vi "SID_mem_to_filter.vi"(11 "mem":u8[](array[numeric]) format="%02x") -> (2 "filter reg":T1 {"vol" format="%0.2f"; "res" format="%0.2f"; "freq" format="%0.2f"})   [LabVIEW 2018]
uses:
  SID_filter_reg.ctl
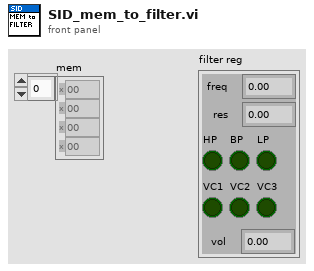
[diagram p1: front panel]
types:
  T1 = typedef "SID_filter_reg.ctl" = cluster{"freq":dbl, "res":dbl, "HP":bool, "BP":bool, "LP":bool, "VC1":bool, "VC2":bool, "VC3":bool, "vol":dbl}
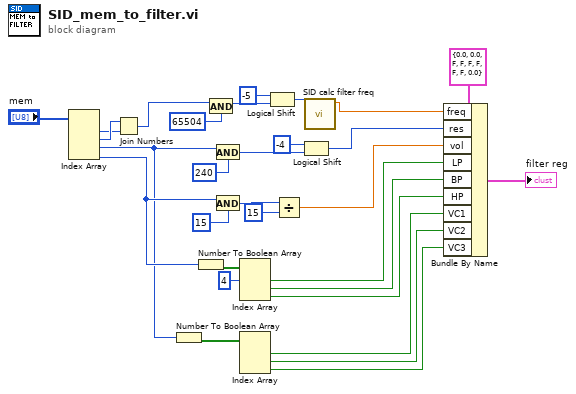
[diagram p0: block diagram]
diagram:
  n1 = Index Array(array="mem") -> (element #1=w7:u8, element #2=w8:u8, element #3=w9:u8, element #4=w10:u8)  [unwired: 4 in]
  n2 = Join Numbers(hi=w8, lo=w7) -> ((hi.lo)=w6:u16)
  n3 = Number To Boolean Array(number=w9) -> (Boolean array=w1:bool[])
  n4 = Number To Boolean Array(number=w10) -> (Boolean array=w23:bool[])
  n5 = And(x=w6, y=u16 65504) -> (x .and. y?=w15:u16)
  n6 = And(x=w9, y=u8 240) -> (x .and. y?=w3:u8)
  n7 = And(x=w10, y=u8 15) -> (x .and. y?=w25:u8)
  n8 = Index Array(array=w23, index #1=4 ("index")) -> (element #1=w21:bool, element #2=w20:bool, element #3=w19:bool)  [unwired: 2 in]
  n9 = Index Array(array=w1) -> (element #1=w18:bool, element #2=w17:bool, element #3=w16:bool)  [unwired: 3 in]
  n10 = Logical Shift(y=i16 -5, x=w15) -> (x << y=w13:u16)
  n11 = Divide(x=w25, y=15) -> (x/y=w24:dbl)
  n12 = Logical Shift(y=i16 -4, x=w3) -> (x << y=w2:u8)
  n13 = call "SID calc filter freq.vi"("x value"=w13) -> ("interpolation value"=w5:dbl)  [unwired: 10 in]
  n14 = Bundle By Name(cluster=T1 {"freq"=0.0, "res"=0.0, "HP"=FALSE, "BP"=FALSE, "LP"=FALSE, "VC1"=FALSE, "VC2"=FALSE, "VC3"=FALSE, "vol"=0.0} ("filter reg"), "freq"=w5, "res"=w2, "vol"=w24, "LP"=w21, "BP"=w20, "HP"=w19, "VC1"=w18, "VC2"=w17, "VC3"=w16) -> (→"filter reg":T1)
